vi "VisionExecute.v.vi"   [LabVIEW 2023]
uses:
  <vilib>/Rock Robotics/WPI/ThirdParty/JAS_Junk/TrajLib/Trajectory_Library.lvlib
  <vilib>/Rock Robotics/WPI/ThirdParty/PhotonVisionLib/PhotonVisionLib.lvlib
  <vilib>/Rock Robotics/WPI/ThirdParty/PhotonPoseStrategy_ENUM.ctl
  VisionGlobal.vi
  <vilib>/Rock Robotics/WPI/ThirdParty/JAS_Junk/TrajLib/TypeDef/TRANSLATION2D.ctl
  <vilib>/Rock Robotics/WPI/ThirdParty/JAS_Junk/TrajLib/TypeDef/ROTATION2D.ctl
  <vilib>/Rock Robotics/WPI/ThirdParty/JAS_Junk/TrajLib/TypeDef/POSE2D.ctl
types:
  T1 = typedef "PhotonVisionLib.lvlib/PhotonPoseStrategy_ENUM.ctl" = enum16{"LOWEST_AMBIGUITY", "CLOSEST_TO_CAMERA_HEIGHT", "CLOSEST_TO_REFERENCE_POSE", "CLOSEST_TO_LAST_POSE", "AVERAGE_BEST_TARGETS", "MULTI_TAG_PNP_ON_COPROCESSOR", "MULTI_TAG_PNP_ON_RIO"}
  T2 = typedef "Trajectory_Library.lvlib/TRANSLATION3D.ctl" = cluster{"X":dbl, "Y":dbl, "Z":dbl}
  T3 = typedef "Trajectory_Library.lvlib/ROTATION3D.ctl" = cluster{"Q_quaternion":T4}
  T4 = typedef "Trajectory_Library.lvlib/QUATERNION.ctl" = cluster{"R":dbl, "V":dbl[]}
  T5 = typedef "Trajectory_Library.lvlib/TRANSFORM3D.ctl" = cluster{"TRANSLATION3D":T2, "ROTATION3D":T3, "XF":bool}
  T6 = typedef "PhotonVisionLib.lvlib/PhotonPipelineResultType.ctl" = cluster{"TargetCount":i32, "Latency_MilliSec":dbl, "Targets":T7[], "TimeStampSec":dbl, "PhotonMultiTargetPNPResult":T9}
  T7 = typedef "PhotonVisionLib.lvlib/PhotonTrackedTargetType.ctl" = cluster{"Yaw":dbl, "Pitch":dbl, "Area":dbl, "Skew":dbl, "MinAreaRectCorners":T8[], "BestCameraToTarget":T5, "FiiducialId":i32, "AltCameraToTarget":T5, "PoseAmbiguity":dbl, "DetectedCorners":T8[]}
  T8 = typedef "PhotonVisionLib.lvlib/TargetCornerType.ctl" = cluster{"X":dbl, "Y":dbl}
  T9 = typedef "PhotonVisionLib.lvlib/PhotonMultiTargetPNPResultType.ctl" = cluster{"PhotonPNPResult":T10, "FiducialIDsUsed":i16[]}
  T10 = typedef "PhotonVisionLib.lvlib/PhotonPNPResultType.ctl" = cluster{"IsPresent":bool, "bestReprojErr":dbl, "altReprojErr":dbl, "ambiguity":dbl, "Best":T5, "Alt":T5}
  T11 = typedef "PhotonVisionLib.lvlib/PhotonPoseEstimator_Configuration.ctl" = cluster{"Primary Strategy":T1, "Camera":string, "Initial Pose":T12, "HighestAmbiguity":dbl, "Use Custom Field":bool, "Custom AprilTag Field":T13, "RobotToCamera":T5, "FallBack Strategy":T1, "BaseNTName":string, "AprilTagField":enum16{"2022 Rapid React", "2023 Charged Up", "2024 Crescendo"}}
  T12 = typedef "Trajectory_Library.lvlib/POSE3D.ctl" = cluster{"Translation3d":T2, "Rotation3d":T3}
  T13 = typedef "Trajectory_Library.lvlib/AprilTagFieldLayout.ctl" = cluster{"AprilTagMap":map{i32, T14}, "FieldLength":dbl, "FieldWidth":dbl, "OriginPosition ":T15, "OriginPose3d":T12}
  T14 = typedef "Trajectory_Library.lvlib/AprilTag.ctl" = cluster{"ID":i32, "POSE3D":T12}
  T15 = typedef "Trajectory_Library.lvlib/AprilTagFieldLayoutOrignPosition_ENUM.ctl" = enum16{"kBlueAllianceWallRightSide,", "kRedAllianceWallRightSide,"}
  T16 = typedef "PhotonVisionLib.lvlib/PhotonEstimatedRobotPoseType.ctl" = cluster{"EstimatedPose":T12, "TimeStamp_Seconds":dbl, "targetsUsed":T7[], "Strategy":T1}
  T17 = typedef "Trajectory_Library.lvlib/POSE2D.ctl" = cluster{"TRANSLATION":T18, "ROTATION":T19}
  T18 = typedef "Trajectory_Library.lvlib/TRANSLATION2D.ctl" = cluster{"X":dbl, "Y":dbl}
  T19 = typedef "Trajectory_Library.lvlib/ROTATION2D.ctl" = cluster{"VALUE":dbl, "COS":dbl, "SIN":dbl}
  T20 = typedef "Trajectory_Library.lvlib/SWERVE_DRIVE_KINEMATICS.ctl" = cluster{"NumModules":i32, "InverseKinematics":T21, "ForwardKinematics":T21, "Modules":T18[], "PrevCoR":T18, "SavedModuleStates":T22[]}
  T21 = typedef "NI_Matrix.lvlib/RealMatrix.ctl" = dbl[][]
  T22 = typedef "Trajectory_Library.lvlib/SWERVE_DRIVE_MODULE_STATE.ctl" = cluster{"Speed":dbl, "Angle":T19}
  T23 = typedef "Trajectory_Library.lvlib/SWERVE_DRIVE_MODULE_POSITION.ctl" = cluster{"Distance":dbl, "Angle":T19, "P":bool}
  T24 = typedef "Trajectory_Library.lvlib/SWERVE_DRIVE_POSE_EST2_CONFIG.ctl" = cluster{"Wheel_Locations M":T18[], "Odom X std dev M":dbl, "Odom Y std dev M":dbl, "Odom Heading std dev Rad":dbl, "Vision X std dev M":dbl, "Vision Y std dev M":dbl, "Vision Heading std dev Rad":dbl}
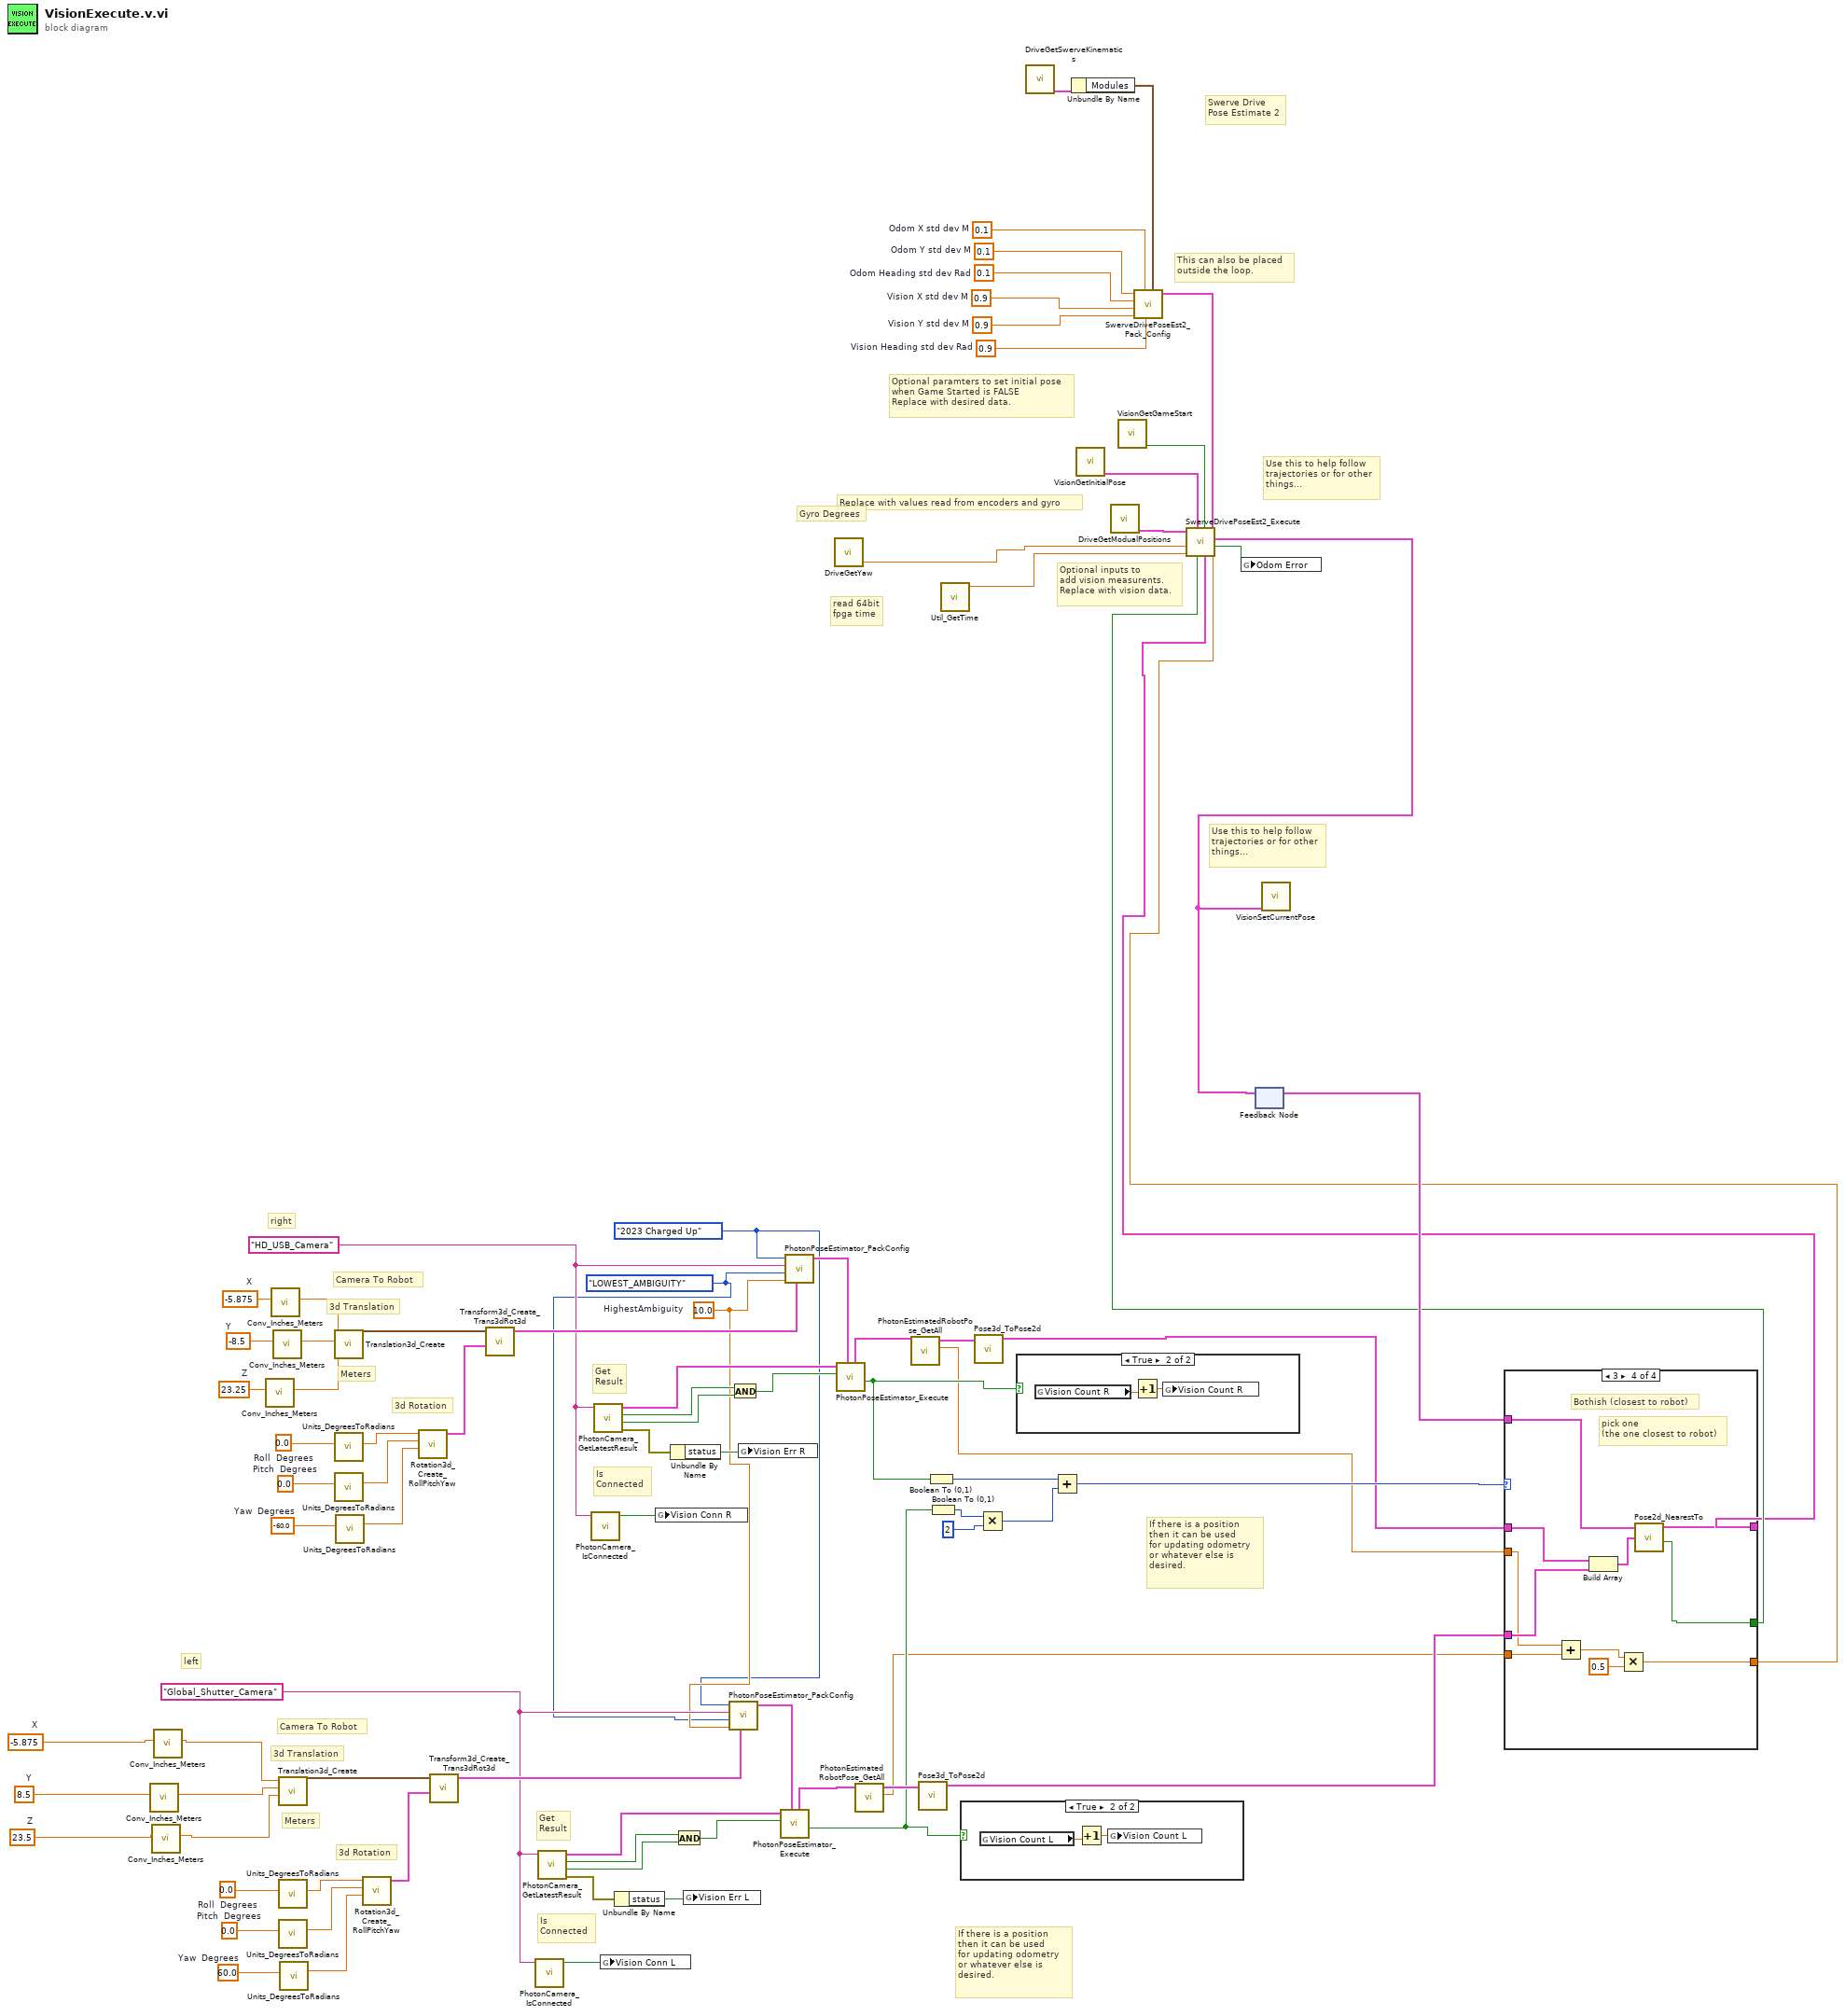
[diagram p0: block diagram]
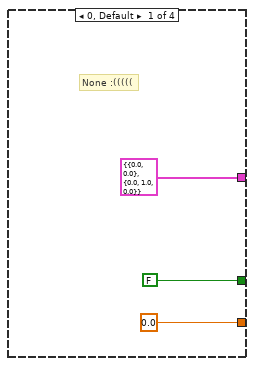
[diagram p2: hidden frame]
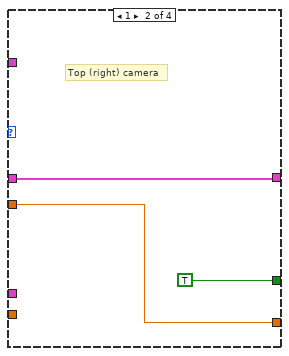
[diagram p3: hidden frame]
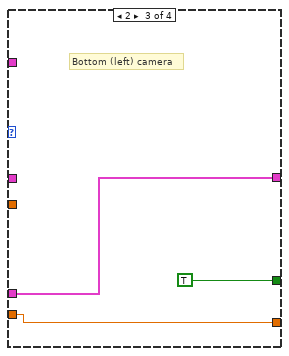
[diagram p4: hidden frame]
diagram:
  w18 = 0.1  # Odom Y std dev M
  w19 = 0.1  # Odom Heading std dev Rad
  w20 = 0.9  # Vision X std dev M
  w21 = 0.9  # Vision Y std dev M
  w22 = 0.1  # Odom X std dev M
  w23 = 0.9  # Vision Heading std dev Rad
  w60 = 0.0  # Roll  Degrees
  w59 = 0.0  # Pitch  Degrees
  w58 = 60.0  # Yaw  Degrees
  w44 = 23.5  # Z
  w48 = -5.875  # X
  w46 = 8.5  # Y
  w54 = "Global_Shutter_Camera" ("CameraName")
  w79 = 0.0  # Roll  Degrees
  w78 = 0.0  # Pitch  Degrees
  w77 = -60.0  # Yaw  Degrees
  w38 = 23.25  # Z
  w42 = -5.875  # X
  w40 = -8.5  # Y
  w36 = 10.0  # HighestAmbiguity
  w35 = PhotonPoseStrategy_ENUM."LOWEST_AMBIGUITY" ("Strategy")
  w34 = enum16{"2022 Rapid React", "2023 Charged Up"}."2023 Charged Up" ("AprilTagField")
  w73 = "HD_USB_Camera" ("CameraName")
  # "Optional inputs to\nadd vision measurents.\nReplace with vision data."
  # "Replace with values read from encoders and gyro"
  # "Optional paramters to set initial pose\nwhen Game Started is FALSE\nReplace with desired data."
  # "read 64bit\nfpga time"
  # "This can also be placed \noutside the loop."
  # "Use this to help follow\ntrajectories or for other\nthings..."
  # "Swerve Drive \nPose Estimate 2"
  # "Use this to help follow\ntrajectories or for other\nthings..."
  # "right"
  # "left"
  # "If there is a position\nthen it can be used\nfor updating odometry\nor whatever else is \ndesired."
  # "Meters"
  # "Camera To Robot"
  # "3d Rotation"
  # "3d Translation"
  # "Is\nConnected"
  # "Get\nResult"
  # "If there is a position\nthen it can be used\nfor updating odometry\nor whatever else is \ndesired."
  # "Meters"
  # "Camera To Robot"
  # "3d Rotation"
  # "3d Translation"
  # "Is\nConnected"
  # "Get\nResult"
  # "Gyro Degrees"
  n1 = call <vilib>:"Conv_Inches_Meters.vi"("INCH"=w46) -> ("Meters"=w45:dbl)  [unwired: 10 in]
  n2 = call <vilib>:"Conv_Inches_Meters.vi"("INCH"=w44) -> ("Meters"=w43:dbl)  [unwired: 10 in]
  n3 = call <vilib>:"Conv_Inches_Meters.vi"("INCH"=w48) -> ("Meters"=w47:dbl)  [unwired: 10 in]
  n4 = call <vilib>:"Conv_Inches_Meters.vi"("INCH"=w38) -> ("Meters"=w37:dbl)  [unwired: 10 in]
  n5 = call <vilib>:"Conv_Inches_Meters.vi"("INCH"=w42) -> ("Meters"=w41:dbl)  [unwired: 10 in]
  n6 = call <vilib>:"Conv_Inches_Meters.vi"("INCH"=w40) -> ("Meters"=w39:dbl)  [unwired: 10 in]
  n7 = call <vilib>:"Translation3d_Create.vi"("Z"=w43, "Y"=w45, "X"=w47) -> ("TRANSLATION3D"=w61:T2)  [unwired: 8 in]
  n8 = call <vilib>:"Units_DegreesToRadians.vi"("Degrees"=w60) -> ("Radians"=w57:dbl)  [unwired: 10 in]
  n9 = call <vilib>:"Units_DegreesToRadians.vi"("Degrees"=w59) -> ("Radians"=w56:dbl)  [unwired: 10 in]
  n10 = call <vilib>:"Units_DegreesToRadians.vi"("Degrees"=w58) -> ("Radians"=w55:dbl)  [unwired: 10 in]
  n11 = call <vilib>:"Translation3d_Create.vi"("Z"=w37, "Y"=w39, "X"=w41) -> ("TRANSLATION3D"=w80:T2)  [unwired: 8 in]
  n12 = call <vilib>:"Units_DegreesToRadians.vi"("Degrees"=w79) -> ("Radians"=w76:dbl)  [unwired: 10 in]
  n13 = call <vilib>:"Units_DegreesToRadians.vi"("Degrees"=w78) -> ("Radians"=w75:dbl)  [unwired: 10 in]
  n14 = call <vilib>:"Units_DegreesToRadians.vi"("Degrees"=w77) -> ("Radians"=w74:dbl)  [unwired: 10 in]
  n15 = call <vilib>:"Rotation3d_Create_RollPitchYaw.vi"("Yaw"=w55, "Pitch"=w56, "Roll"=w57) -> ("Rotation3d"=w62:T3)  [unwired: 8 in]
  n16 = call <vilib>:"Rotation3d_Create_RollPitchYaw.vi"("Yaw"=w74, "Pitch"=w75, "Roll"=w76) -> ("Rotation3d"=w81:T3)  [unwired: 8 in]
  n17 = call <vilib>:"Transform3d_Create_Trans3dRot3d.vi"("Rotation3d"=w62, "Translation3d"=w61) -> ("Transform3d"=w63:T5)  [unwired: 9 in]
  n18 = call <vilib>:"Transform3d_Create_Trans3dRot3d.vi"("Rotation3d"=w81, "Translation3d"=w80) -> ("Transform3d"=w82:T5)  [unwired: 9 in]
  n19 = call <vilib>:"PhotonCamera_IsConnected.vi"("CameraName"=w54) -> ("IsConnected"=w51:bool)  [unwired: 9 in, 1 out]
  n20 = call <vilib>:"PhotonCamera_GetLatestResult.vi"("CameraName"=w54) -> ("error out"=w50:errorcluster, "New Data"=w67:bool, "HasTargets"=w66:bool, "PipelineResult"=w64:T6)  [unwired: 7 in]
  n21 = call <vilib>:"PhotonCamera_IsConnected.vi"("CameraName"=w73) -> ("IsConnected"=w70:bool)  [unwired: 9 in, 1 out]
  n22 = call <vilib>:"PhotonCamera_GetLatestResult.vi"("CameraName"=w73) -> ("error out"=w69:errorcluster, "New Data"=w86:bool, "HasTargets"=w85:bool, "PipelineResult"=w83:T6)  [unwired: 7 in]
  n23 = global write "VisionGlobal.vi" "Vision Conn L"(w51) -> ()
  n24 = Unbundle By Name(w50) -> ("status"=w49:bool)
  n25 = global write "VisionGlobal.vi" "Vision Conn R"(w70) -> ()
  n26 = Unbundle By Name(w69) -> ("status"=w68:bool)
  n27 = And(x=w66, y=w67) -> (x .and. y?=w65:bool)
  n28 = global write "VisionGlobal.vi" "Vision Err L"(w49) -> ()
  n29 = call <vilib>:"PhotonPoseEstimator_PackConfig.vi"("RobotToCamera"=w63, "HighestAmbiguity"=w36, "PirmaryStrategy"=w35, "Camera"=w54, "AprilTagField"=w34) -> ("PoseEstimator_Configuration"=w53:T11)  [unwired: 6 in]
  n30 = And(x=w85, y=w86) -> (x .and. y?=w84:bool)
  n31 = global write "VisionGlobal.vi" "Vision Err R"(w68) -> ()
  n32 = call <vilib>:"PhotonPoseEstimator_Execute.vi"("Configuration"=w53, "PIpeline Has \nNew Results"=w65, "PipelineResult"=w64) -> ("New Pose Found"=w32:bool, "PhotonEstimatedRobotPose"=w3:T16)  [unwired: 3 in, 4 out]
  n33 = call <vilib>:"PhotonPoseEstimator_PackConfig.vi"("RobotToCamera"=w82, "HighestAmbiguity"=w36, "PirmaryStrategy"=w35, "Camera"=w73, "AprilTagField"=w34) -> ("PoseEstimator_Configuration"=w72:T11)  [unwired: 6 in]
  n34 = call "DriveGetYaw.vi"() -> ("Yaw"=w13:dbl)  [unwired: 11 in]
  n35 = call <vilib>:"PhotonPoseEstimator_Execute.vi"("Configuration"=w72, "PIpeline Has \nNew Results"=w84, "PipelineResult"=w83) -> ("New Pose Found"=w33:bool, "PhotonEstimatedRobotPose"=w4:T16)  [unwired: 3 in, 4 out]
  n36 = call <vilib>:"PhotonEstimatedRobotPose_GetAll.vi"("PhotonEstimatedRobotPose"=w3) -> ("TimeStamp_Seconds"=w2:dbl, "EstimatedPose"=w52:T12)  [unwired: 7 in, 2 out]
  n37 = call <vilib>:"PhotonEstimatedRobotPose_GetAll.vi"("PhotonEstimatedRobotPose"=w4) -> ("TimeStamp_Seconds"=w1:dbl, "EstimatedPose"=w71:T12)  [unwired: 7 in, 2 out]
  n38 = call <vilib>:"Pose3d_ToPose2d.vi"("in Pose3d"=w52) -> ("out Pose2d"=w25:T17)  [unwired: 10 in]
  n39 = Boolean To (0,1)(Boolean=w33) -> (0, 1=w28:i16)
  n40 = Boolean To (0,1)(Boolean=w32) -> (0, 1=w31:i16)
  n41 = call <vilib>:"Util_GetTime.vi"() -> ("FPGA_Time_Seconds"=w10:dbl)  [unwired: 9 in, 2 out]
  n42 = case shown="True" w32 {
    frame False {
    }
    frame True {
      n43 = global read "VisionGlobal.vi" "Vision Count L"() -> (w87:dbl)
      n44 = Increment(x=w87) -> (x+1=w88:dbl)
      n45 = global write "VisionGlobal.vi" "Vision Count L"(w88) -> ()
    }
  }
  n46 = call <vilib>:"Pose3d_ToPose2d.vi"("in Pose3d"=w71) -> ("out Pose2d"=w26:T17)  [unwired: 10 in]
  n47 = Multiply(x=w31, y=i16 2) -> (x*y=w29:i16)
  n48 = case shown="True" w33 {
    frame False {
    }
    frame True {
      n49 = global read "VisionGlobal.vi" "Vision Count R"() -> (w89:dbl)
      n50 = Increment(x=w89) -> (x+1=w90:dbl)
      n51 = global write "VisionGlobal.vi" "Vision Count R"(w90) -> ()
    }
  }
  n52 = call "DriveGetSwerveKinematics.vi"() -> ("SWERVE_DRIVE_KINEMATICS"=w6:T20)  [unwired: 11 in]
  n53 = Add(x=w28, y=w29) -> (x+y=w27:i16)
  n54 = Unbundle By Name(w6) -> ("Modules"=w5:T18[])
  n55 = call "VisionGetInitialPose.vi"() -> ("InitialPose"=w11:T17)  [unwired: 10 in]
  n56 = call "DriveGetModualPositions.vi"() -> ("Swerve_Drive_Modual_Positions"=w14:T23[])  [unwired: 11 in]
  n57 = call "VisionGetGameStart.vi"() -> ("Game Start"=w12:bool)  [unwired: 11 in]
  n58 = call <vilib>:"SwerveDrivePoseEst2_Pack_Config.vi"("Wheel_Locations M"=w5, "Vision Heading std dev Rad"=w23, "Odom X std dev M"=w22, "Vision Y std dev M"=w21, "Vision X std dev M"=w20, "Odom Heading std dev Rad"=w19, "Odom Y std dev M"=w18) -> ("SwervePoseEst2Config"=w17:T24)  [unwired: 4 in]
  n59 = feedback #1() -> (w24:T17)  [unwired: 1 in]
  n60 = case shown="3" w27 {
    tunnel: w26 -> [_ w95 _ w108]
    tunnel: w25 -> [_ _ w98 w107]
    tunnel: w24 -> [_ _ _ w109]
    tunnel: [FALSE ("Found") TRUE ("Found") TRUE ("Found") w105] -> w9
    tunnel: w1 -> [_ w96 _ w104]
    tunnel: w2 -> [_ _ w99 w103]
    tunnel: [T17 {"TRANSLATION"={"X"=0.0, "Y"=0.0}, "ROTATION"={"VALUE"=0.0, "COS"=1.0, "SIN"=0.0}} ("Nearest Pose") w95 w98 w106] -> w8
    tunnel: [0.0 w96 w99 w100] -> w7
    frame 0, Default {
      # "None :((((("
    }
    frame 1 {
      # "Top (right) camera"
    }
    frame 2 {
      # "Bottom (left) camera"
    }
    frame 3 {
      # "pick one \n(the one closest to robot)"
      # "Bothish (closest to robot)"
      n61 = Add(x=w104, y=w103) -> (x+y=w102:dbl)
      n62 = Build Array(w108, w107) -> (w110:T17[])
      n63 = Multiply(x=w102, y=0.5) -> (x*y=w100:dbl)
      n64 = call <vilib>:"Pose2d_NearestTo.vi"("other POSE"=w110, "in POSE"=w109) -> ("Found"=w105:bool, "Nearest Pose"=w106:T17)  [unwired: 8 in]
    }
  }
  n65 = call <vilib>:"SwerveDrivePoseEst2_Execute.vi"("Vision TImeStamp_Seconds"=w7, "SwervePoseEst2Config"=w17, "visionRobotPose"=w8, "Game Started"=w12, "Add Vision Meas"=w9, "InitialPose"=w11, "Pass Through Time"=w10, "Gyro Degrees"=w13, "Module Positions"=w14) -> ("Error"=w15:bool, "Estimated Pose"=w16:T17)  [unwired: 1 in]
  n66 = global write "VisionGlobal.vi" "Odom Error"(w15) -> ()
  n67 = feedback-in #1(w16) -> ()
  n68 = call "VisionSetCurrentPose.vi"("Current Pose"=w16) -> ()  [unwired: 11 in]
